vi "DAQ Assist Output 4.vi"(7 "index":i32) -> ()   [LabVIEW 2015]
panel:
  in  "data":u32[](array[numeric])=[0, 1, 12, 5, 9, 0, 0, 0, 0, 0, 0, 0]
  in  "device name":tag="Dev3"
  in  "error in":errorcluster
  out "error out":errorcluster
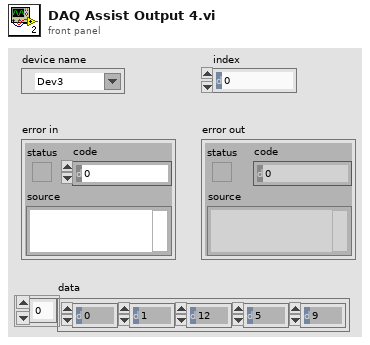
[diagram p1: front panel]
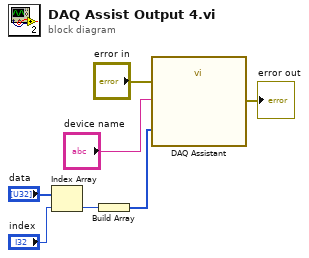
[diagram p0: block diagram]
diagram:
  n1 = Index Array(array="data", index="index") -> (element=w2:u32)
  n2 = Build Array(w2) -> (w1:u32[])
  n3 = call "DAQ Assistant"("data"=w1, "error in"="error in", "device name"="device name") -> ("error out"=→"error out":errorcluster)  [unwired: 15 in, 1 out]
